vi "Display Data to Table.vi"(11 "Macro":T1) -> (1 "Metadata":string, 3 "Macro Steps":string[][](array[string]))   [LabVIEW 2023]
doc: "Converts <B>Macro</B> to a table of macro steps and a string of associated metadata."
uses:
  CTLs/Macro Cluster v2.0.ctl
  CTLs/Step.ctl
  CTLs/Step Type.ctl
panel:
  in  "Virtual Key":u8(ring)=65
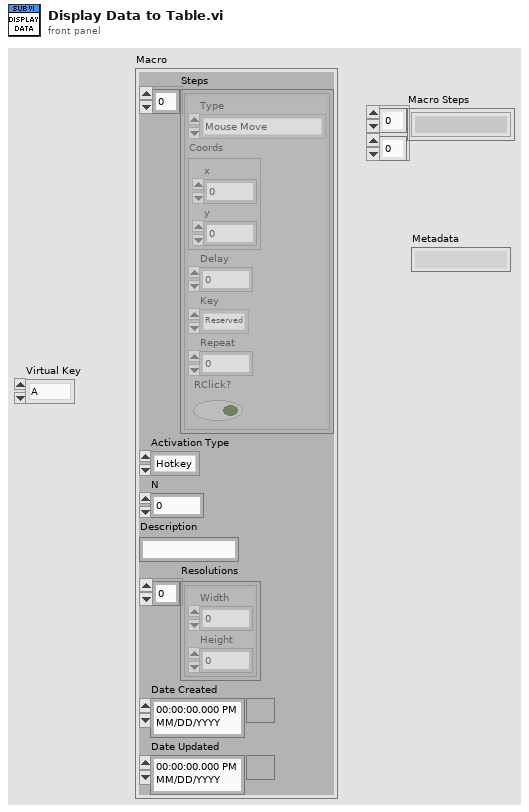
[diagram p1: front panel]
types:
  T1 = typedef "Macro Cluster v2.0.ctl" = cluster{"Steps":T2[], "Activation Type":enum32{"Hotkey", "Automatic"}, "N":i32, "Description":string, "Resolutions":cluster{"Width":i16, "Height":i16}[], "Date Created":timestamp, "Date Updated":timestamp}
  T2 = typedef "Step.ctl" = cluster{"Type":T3, "Coords":cluster{"x":i32, "y":i32}, "Delay":i32, "Key":u8, "Repeat":i32, "RClick?":bool}
  T3 = typedef "Step Type.ctl" = enum16{"Mouse Move", "Mouse Click", "Key Press", "Wait", "Mouse Down", "Mouse Up", "Key Down", "Key Up"}
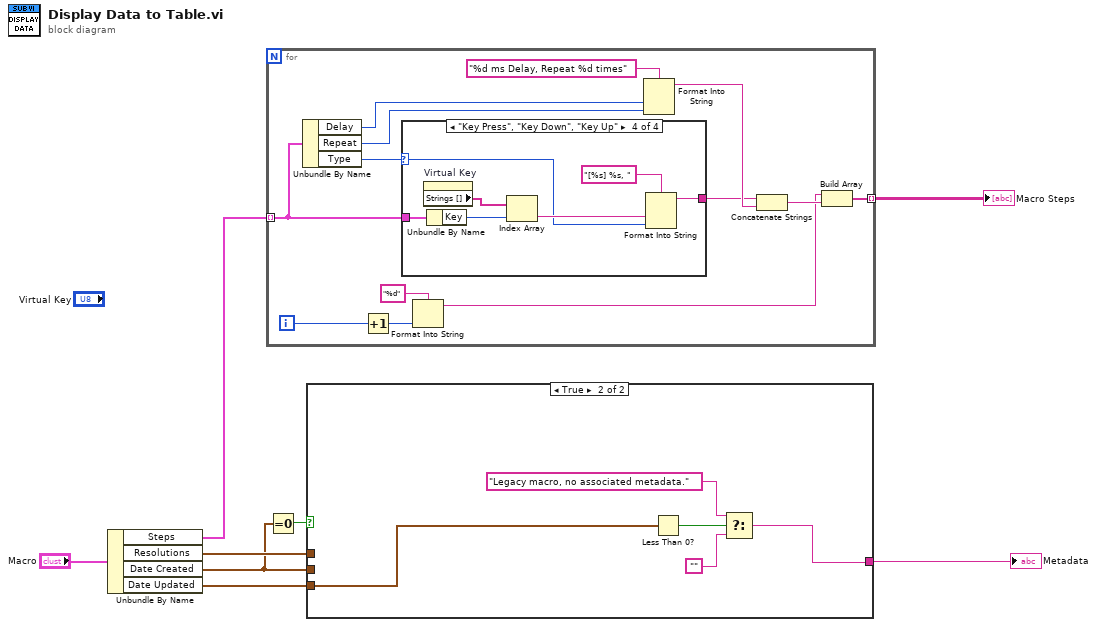
[diagram p0: block diagram]
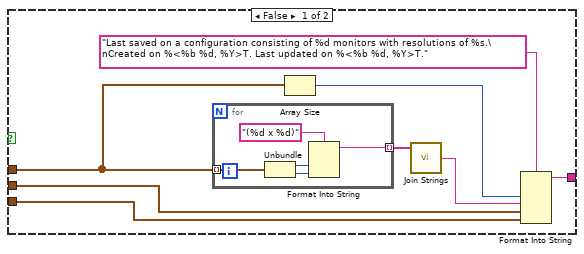
[diagram p2: hidden frame]
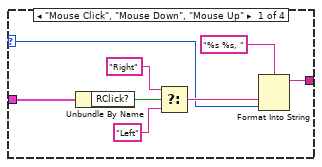
[diagram p3: hidden frame]
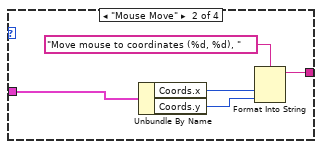
[diagram p4: hidden frame]
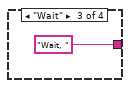
[diagram p5: hidden frame]
diagram:
  n1 = Unbundle By Name("Macro") -> ("Steps"=w6:T2[], "Resolutions"=w4:cluster{"Width":i16, "Height":i16}[], "Date Created"=w1:timestamp, "Date Updated"=w5:timestamp)
  n2 = for {
    tunnel: w6 -> [w17] mode=indexing
    tunnel: [w11] -> w8 mode=indexing
    i -> [w13]
    n3 = Unbundle By Name(w17) -> ("Delay"=w10:i32, "Repeat"=w9:i32, "Type"=w20:T3)
    n4 = Increment(x=w13) -> (x+1=w15:i32)
    n5 = case shown="\"Key Press\", \"Key Down\", \"Key Up\"" w20 {
      selector: w20 -> [w23 _ _ w37]
      tunnel: w17 -> [w25 w34 _ w42]
      tunnel: [w22 w33 "Wait, " w36] -> w19
      frame "Mouse Click", "Mouse Down", "Mouse Up" {
        n6 = Unbundle By Name(w25) -> ("RClick?"=w28:bool)
        n7 = Select(t="Right", s=w28, f="Left") -> (s? t:f=w24:string)
        n8 = Format Into String(format string="%s %s, ", w24, w23) -> (resulting string=w22:string)  [unwired: 2 in, 1 out]
      }
      frame "Mouse Move" {
        n9 = Unbundle By Name(w34) -> ("Coords.x"=w31:i32, "Coords.y"=w30:i32)
        n10 = Format Into String(format string="Move mouse to coordinates (%d, %d), ", w31, w30) -> (resulting string=w33:string)  [unwired: 2 in, 1 out]
      }
      frame "Wait" {
      }
      frame "Key Press", "Key Down", "Key Up" {
        n11 = property on="Virtual Key" class="Ring (strict)"() -> ("Strings []"=w40:string[])  [unwired: 2 in, 2 out]
        n12 = Unbundle By Name(w42) -> ("Key"=w39:u8)
        n13 = Index Array(array=w40, index=w39) -> (element=w38:string)
        n14 = Format Into String(format string="[%s] %s, ", w38, w37) -> (resulting string=w36:string)  [unwired: 2 in, 1 out]
      }
    }
    n15 = Format Into String(format string="%d", w15) -> (resulting string=w12:string)  [unwired: 2 in, 1 out]
    n16 = Format Into String(format string="%d ms Delay, Repeat %d times", w10, w9) -> (resulting string=w21:string)  [unwired: 2 in, 1 out]
    n17 = Concatenate Strings(w19, w21) -> (w16:string)
    n18 = Build Array(w12, w16) -> (w11:string[])
  }
  "Macro Steps" <- w8
  n19 = Equal To 0?(x=w1) -> (x = 0?=w2:bool)
  n20 = case shown="True" w2 {
    tunnel: w5 -> [w49 w60]
    tunnel: w1 -> [w48 _]
    tunnel: w4 -> [w46 _]
    tunnel: [w43 w56] -> w3
    frame False {
      n21 = for {
        tunnel: w46 -> [w54] mode=indexing
        tunnel: [w51] -> w45 mode=indexing
        n22 = Unbundle(w54) -> ("Width"=w52:i16, "Height"=w53:i16)
        n23 = Format Into String(format string="(%d x %d)", w52, w53) -> (resulting string=w51:string)  [unwired: 2 in, 1 out]
      }
      n24 = Array Size(array=w46) -> (size(s)=w47:i32)
      n25 = call <vilib>:"Join Strings.vi"("Strings In"=w45) -> ("String"=w44:string)  [unwired: 2 in]
      n26 = Format Into String(format string="Last saved on a configuration consisting of %d monitors with resolutions of %s.\nCreated on %<%b %d, %Y>T. Last updated on %<%b %d, %Y>T.", w47, w44, w48, w49) -> (resulting string=w43:string)  [unwired: 2 in, 1 out]
    }
    frame True {
      n27 = Less Than 0?(x=w60) -> (x < 0?=w59:bool)
      n28 = Select(t="Legacy macro, no associated metadata.", s=w59, f="") -> (s? t:f=w56:string)
    }
  }
  "Metadata" <- w3
